vi "Tx Buffered Packet Page.vi"(8 "error in (no error)":errorcluster, 11 "Node Ptr":T5 format="%.0x") -> (0 "error out":errorcluster)   [LabVIEW 2016, in "UDP-Custom-Device System Explorer.lvlib"]
uses:
  UDP-Custom-Device System Explorer.lvlib
  Shared/Types/Shared - Transmit Flag Options.ctl
  Shared/Types/Shared - Pointer Encoding.ctl
  <vilib>/NI Veristand/Custom Device API/Custom Device Item Ref.ctl
  Shared/Types/Shared - Buffer Options.ctl
  Shared/Types/Shared - Transmit Echo Options.ctl
  Types/Page References/Refs - Tx Buffered Data Packet Page.ctl
  <vilib>/NI VeriStand/Custom Device API/Custom Device API.lvlib
  Property Accessors/Shared Packet Accessors.lvlib
  Property Accessors/Tx Packet Accessors.lvlib
  Property Accessors/Buffered Data Packet.lvlib
  Shared/UDP-Custom-Device Shared.lvlib
panel:
  in  "Debug Mode":bool caption="Auto-Assign Local NIC"
  in  "Transmit Echo Options":T1
  in  "Buffer Options":T2
  in  "Transmit Options":T3=enum."One-Shot"
  in  "Port as Channel?":bool caption="Auto-Assign Local NIC"
  in  "Pointer Encoding":T4
  in  "TTL":u16=1
  in  "Multicast?":bool caption="Auto-Assign Local NIC"
  in  "External Buffer?":bool
  in  "Buffer Size (bytes)":u32
  in  "General Header 3":cluster{"Section Name":string}={"Section Name"="Buffer Configuration"}
  in  "Prepend\nHeader?":bool caption="Auto-Assign Local NIC"
  in  "Auto-Assign Local NIC":bool
  in  "Port":u16
  in  "IP Address of Local NIC":string
  in  "Decimation":u16
  in  "General Header 2":cluster{"Section Name":string}={"Section Name"="Network Settings"}
  in  "Destination Port":u16
  in  "IP Address of Destination":string
  in  "Configure Header":bool
  in  "Endianness":u16(ring) items=["big-endian"=0, "little-endian"=2]
  out "Packet ID":i32
  in  "Description":string
  in  "Name":string
  in  "SHDocVw.IWebBrowser":refnum<k7>(container)
  in  "General Header":cluster{"Section Name":string}={"Section Name"="Buffered Transmit Packet"}
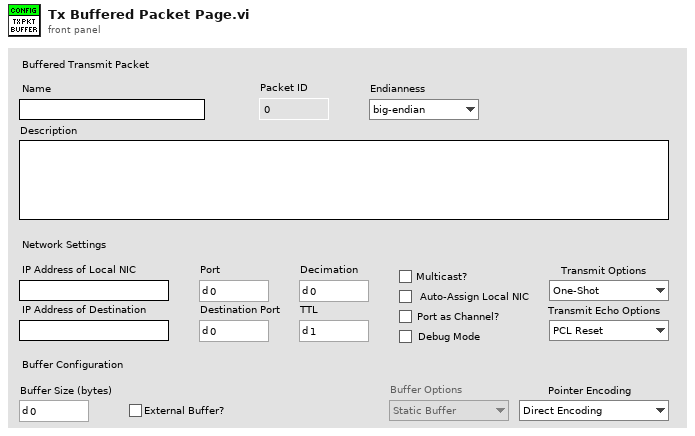
[diagram p1: front panel]
types:
  T1 = typedef "UDP-Custom-Device Shared.lvlib/Shared - Transmit Echo Options.ctl" = enum16{"PCL Reset", "Counter", "Mirror"}
  T2 = typedef "UDP-Custom-Device Shared.lvlib/Shared - Buffer Options.ctl" = enum16{"Static Buffer", "Circular Buffer"}
  T3 = typedef "UDP-Custom-Device Shared.lvlib/Shared - Transmit Flag Options.ctl" = enum16{"Always", "One-Shot", "Toggle"}
  T4 = typedef "UDP-Custom-Device Shared.lvlib/Shared - Pointer Encoding.ctl" = enum16{"Direct Encoding", "Conversion Encoding"}
  T5 = typedef "Custom Device API.lvlib/Custom Device Item Ref.ctl" = u64
  T6 = typedef "UDP-Custom-Device System Explorer.lvlib/Refs - Tx Buffered Data Packet Page.ctl" = cluster{"Name":refnum<vi>, "Description":refnum<vi>, "Packet ID":refnum<vi>, "Endianness":refnum<vi>, "Prepend\nHeader?":refnum<vi>, "Configure Header":refnum<vi>, "Decimation":refnum<vi>, "IP Address of Local NIC":refnum<vi>, "Port":refnum<vi>, "IP Address of Destination":refnum<vi>, "Destination Port":refnum<vi>, "Auto-Assign Local NIC":refnum<vi>, "External Buffer?":refnum<vi>, "Buffer Size (bytes)":refnum<vi>, "Multicast?":refnum<vi>, "TTL":refnum<vi>, "Pointer Encoding":refnum<vi>, "Port as Channel?":refnum<vi>, "Transmit Options":refnum<vi>, "Buffer Options":refnum<vi>, "Transmit Echo Options":refnum<vi>, "Debug Mode":refnum<vi>}
  T7 = enum8{"Enabled", "Disabled", "Disabled and Grayed Out"}
  T8 = typedef "Custom Device API.lvlib/Custom Device Commands.ctl" = enum16{"Default", "Item renamed", "Shutdown", "Dynamic button pressed"}
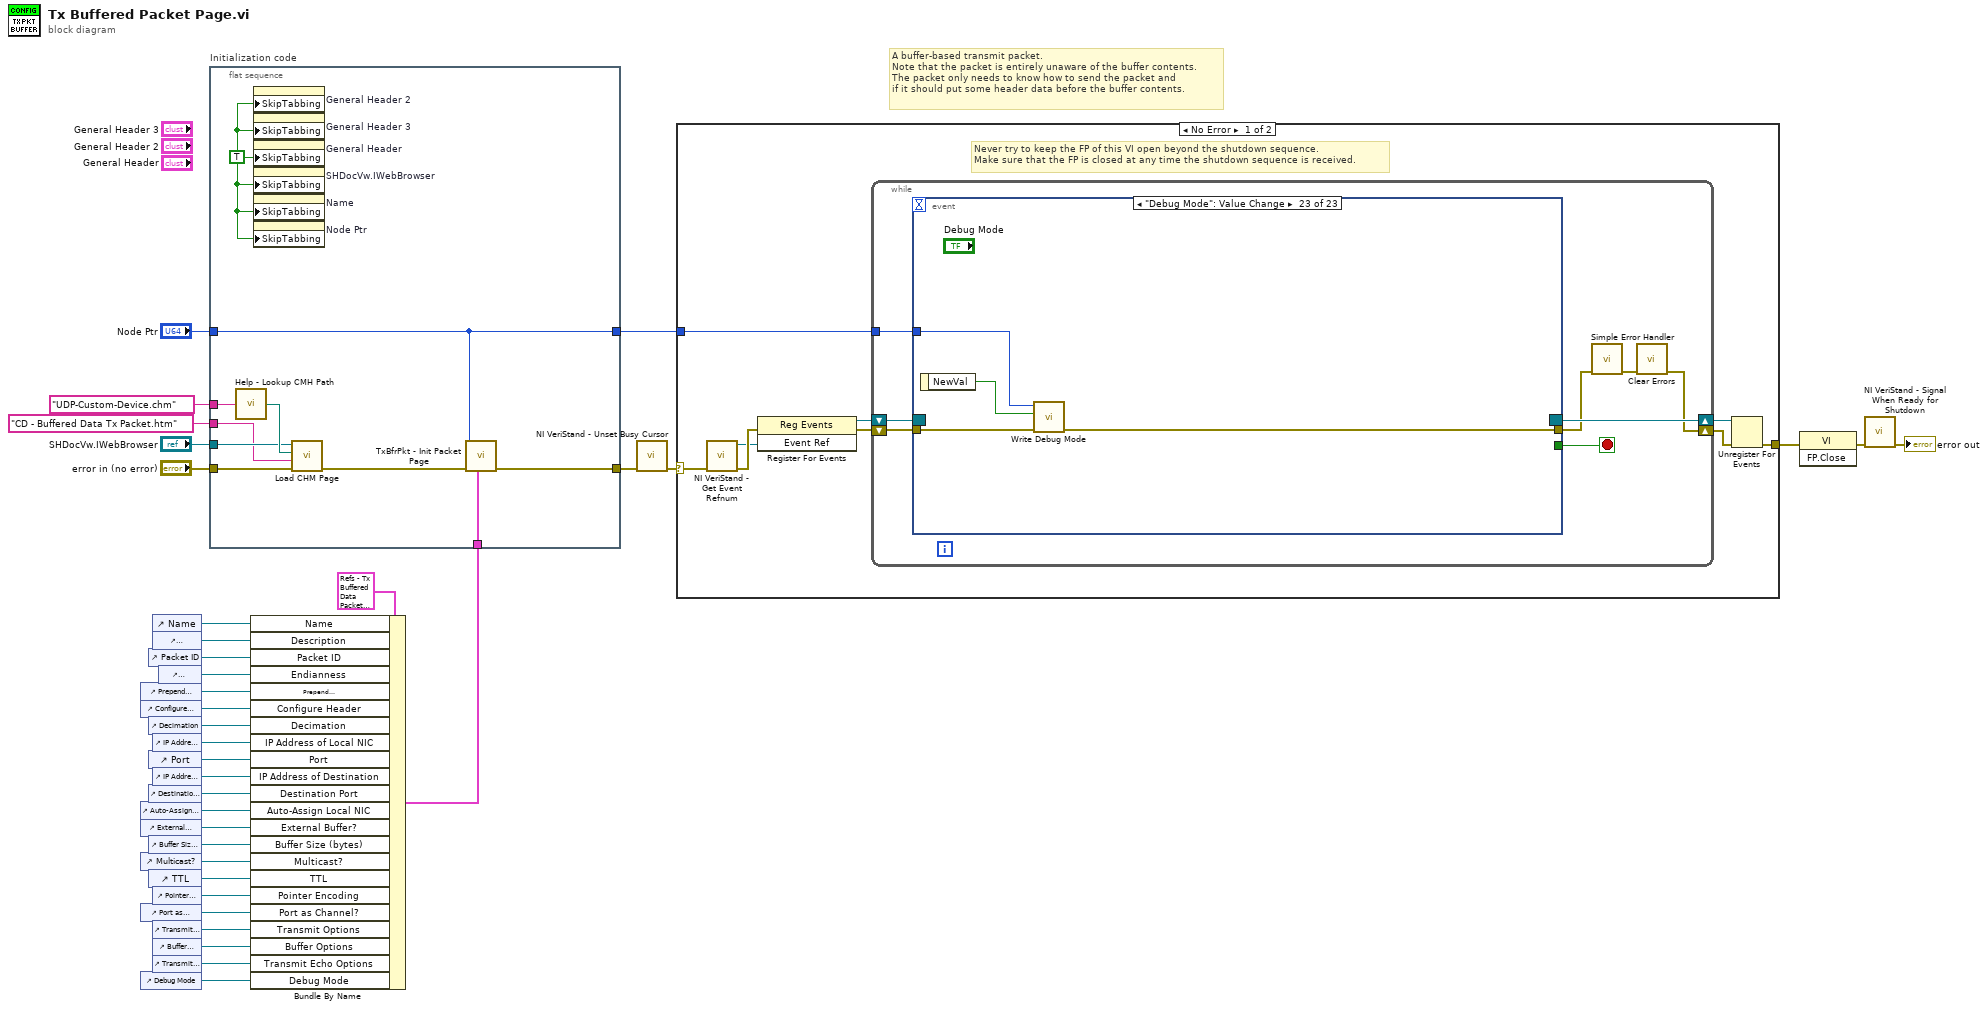
[diagram p0: block diagram]
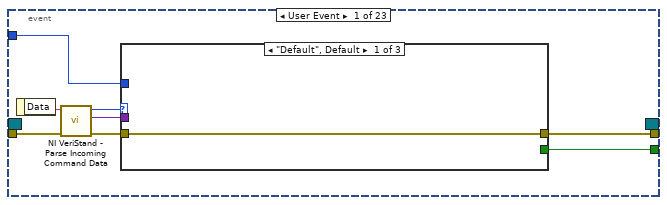
[diagram p2: hidden frame]
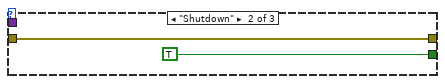
[diagram p3: hidden frame]
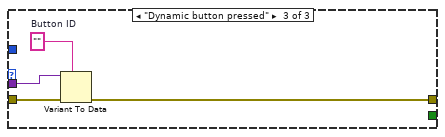
[diagram p4: hidden frame]
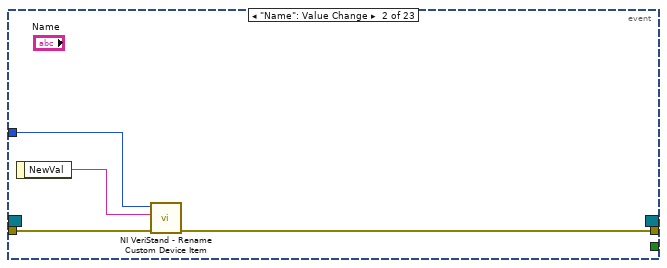
[diagram p5: hidden frame]
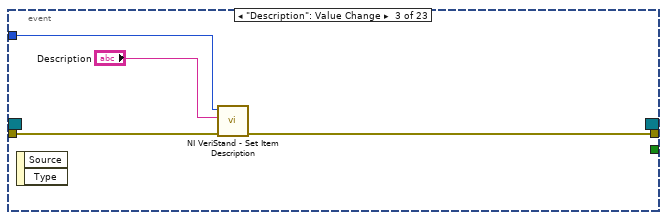
[diagram p6: hidden frame]
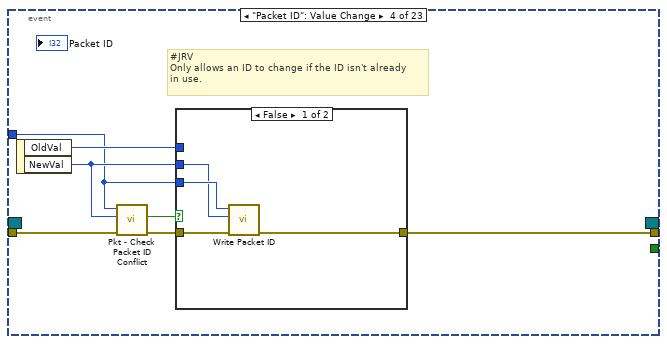
[diagram p7: hidden frame]
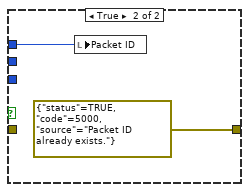
[diagram p8: hidden frame]
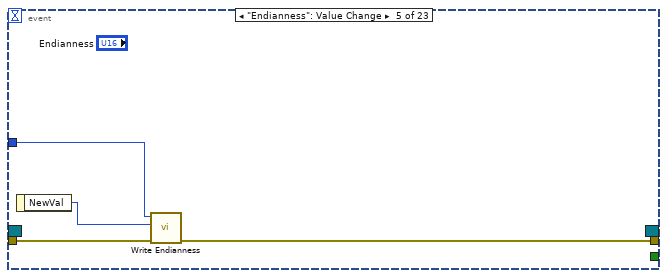
[diagram p9: hidden frame]
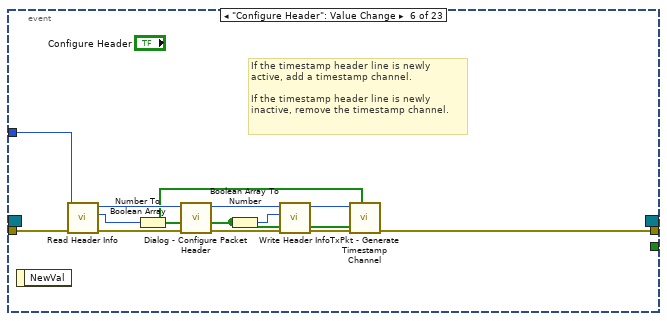
[diagram p10: hidden frame]
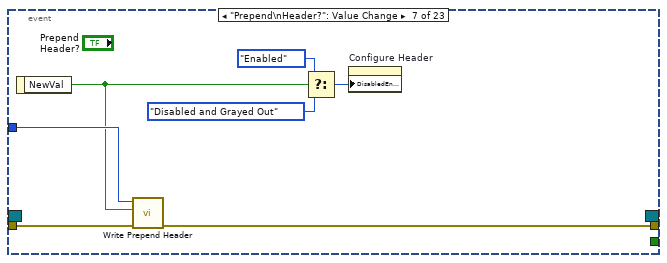
[diagram p11: hidden frame]
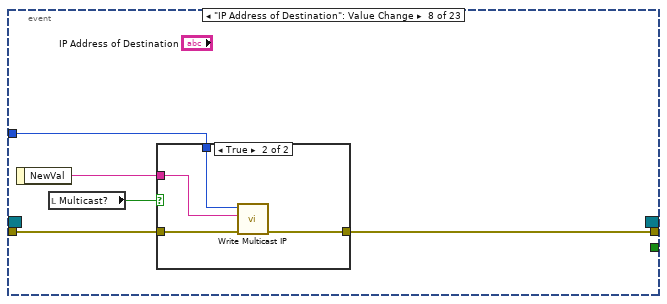
[diagram p12: hidden frame]
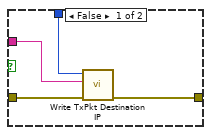
[diagram p13: hidden frame]
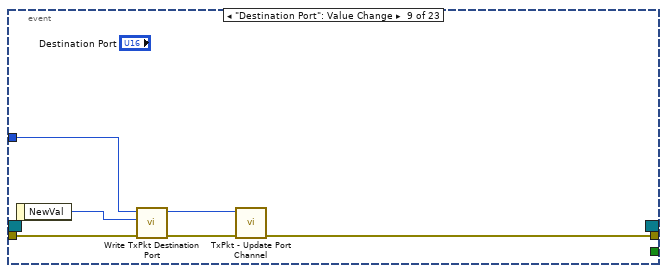
[diagram p14: hidden frame]
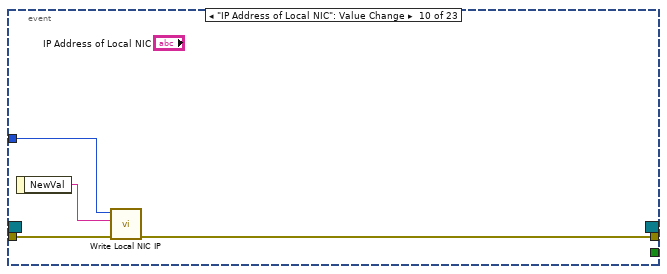
[diagram p15: hidden frame]
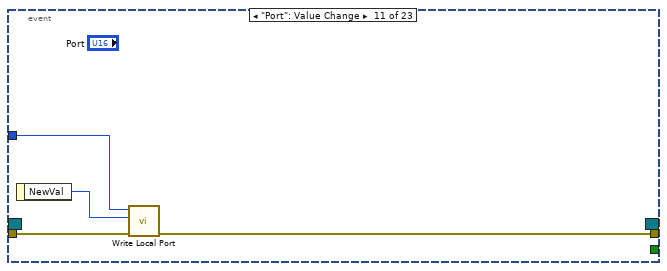
[diagram p16: hidden frame]
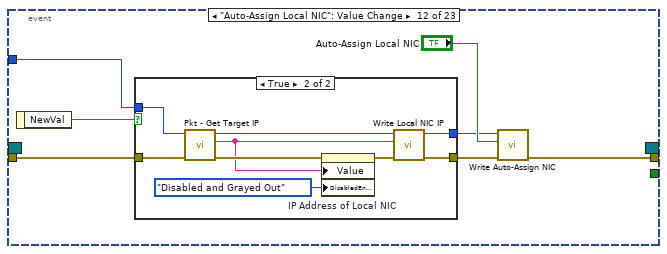
[diagram p17: hidden frame]
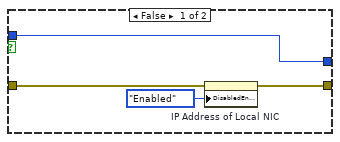
[diagram p18: hidden frame]
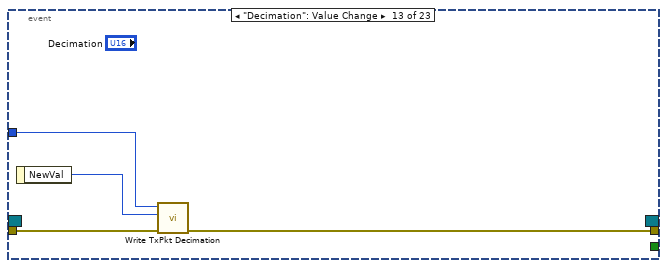
[diagram p19: hidden frame]
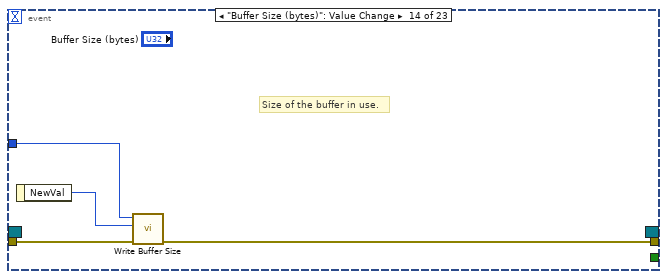
[diagram p20: hidden frame]
diagram:
  # "A buffer-based transmit packet.\nNote that the packet is entirely unaware of the buffer contents.\nThe packet only needs to know how to send the packet and\nif it should put some header data before the buffer contents."
  n1 = control-ref of="Prepend\nHeader?"() -> (w19:refnum<vi>)
  n2 = control-ref of="Configure Header"() -> (w18:refnum<vi>)
  n3 = control-ref of="Auto-Assign Local NIC"() -> (w12:refnum<vi>)
  n4 = control-ref of="External Buffer?"() -> (w11:refnum<vi>)
  n5 = control-ref of="Multicast?"() -> (w8:refnum<vi>)
  n6 = control-ref of="Port as Channel?"() -> (w5:refnum<vi>)
  n7 = control-ref of="Debug Mode"() -> (w1:refnum<vi>)
  n8 = control-ref of="Packet ID"() -> (w21:refnum<vi>)
  n9 = control-ref of="Decimation"() -> (w17:refnum<vi>)
  n10 = control-ref of="Port"() -> (w15:refnum<vi>)
  n11 = control-ref of="Destination Port"() -> (w13:refnum<vi>)
  n12 = control-ref of="Buffer Size (bytes)"() -> (w10:refnum<vi>)
  n13 = control-ref of="TTL"() -> (w7:refnum<vi>)
  n14 = control-ref of="Name"() -> (w23:refnum<vi>)
  n15 = control-ref of="Description"() -> (w22:refnum<vi>)
  n16 = control-ref of="IP Address of Local NIC"() -> (w16:refnum<vi>)
  n17 = control-ref of="IP Address of Destination"() -> (w14:refnum<vi>)
  n18 = control-ref of="Pointer Encoding"() -> (w6:refnum<vi>)
  n19 = control-ref of="Transmit Options"() -> (w4:refnum<vi>)
  n20 = control-ref of="Buffer Options"() -> (w3:refnum<vi>)
  n21 = control-ref of="Transmit Echo Options"() -> (w2:refnum<vi>)
  n22 = control-ref of="Endianness"() -> (w20:refnum<vi>)
  n23 = flat-sequence "Initialization code" {
    tunnel: "error in (no error)" -> [w44]
    tunnel: "Node Ptr" -> [w39]
    tunnel: [w37] -> w31
    tunnel: [w39] -> w28
    tunnel: "SHDocVw.IWebBrowser" -> [w43]
    tunnel: "CD - Buffered Data Tx Packet.htm" ("CD_CHM_Section") -> [w41]
    tunnel: "UDP-Custom-Device.chm" ("CD_CHM_FileName") -> [w42]
    tunnel: w9 -> [w36]
    frame #0 {
      w40 = TRUE ("Skip When Tabbing")
      n24 = call "Help - Lookup CMH Path.vi"("Main CMH File"=w42) -> ("Compiled CMH Path"=w45:path)
      n25 = property on="General Header 2" class="Clust (strict)"("SkipTabbing"=w40) -> ()  [unwired: 2 in, 2 out]
      n26 = property on="General Header 3" class="Clust (strict)"("SkipTabbing"=w40) -> ()  [unwired: 2 in, 2 out]
      n27 = property on="General Header" class="Clust (strict)"("SkipTabbing"=w40) -> ()  [unwired: 2 in, 2 out]
      n28 = property on="SHDocVw.IWebBrowser" class="AXCont"("SkipTabbing"=w40) -> ()  [unwired: 2 in, 2 out]
      n29 = property on="Name" class="Str"("SkipTabbing"=w40) -> ()  [unwired: 2 in, 2 out]
      n30 = property on="Node Ptr" class="DigNum (strict)"("SkipTabbing"=w40) -> ()  [unwired: 2 in, 2 out]
      n31 = call <vilib>:"Load CHM Page.vi"("error in (no error)"=w44, "HTML File"=w41, "Compiled CHM Path"=w45, "Web Browser Reference"=w43) -> ("error out"=w38:errorcluster)  [unwired: 7 in]
      n32 = call "TxBfrPkt - Init Packet Page.vi"("Tx Buffered Data Packet Refs"=w36, "error in (no error)"=w38, "Node Ptr In"=w39) -> ("error out"=w37:errorcluster)  [unwired: 7 in, 1 out]
    }
  }
  n33 = Bundle By Name(cluster=T6 {"Name"=refnum, "Description"=refnum, "Packet ID"=refnum, "Endianness"=refnum, "Prepend\nHeader?"=refnum, "Configure Header"=refnum, "Decimation"=refnum, "IP Address of Local NIC"=refnum, "Port"=refnum, "IP Address of Destination"=refnum, "Destination Port"=refnum, "Auto-Assign Local NIC"=refnum, "External Buffer?"=refnum, "Buffer Size (bytes)"=refnum, "Multicast?"=refnum, "TTL"=refnum, "Pointer Encoding"=refnum, "Port as Channel?"=refnum, "Transmit Options"=refnum, "Buffer Options"=refnum, "Transmit Echo Options"=refnum, "Debug Mode"=refnum} ("Tx Buffered Data Packet Refs"), "Name"=w23, "Description"=w22, "Packet ID"=w21, "Endianness"=w20, "Prepend\nHeader?"=w19, "Configure Header"=w18, "Decimation"=w17, "IP Address of Local NIC"=w16, "Port"=w15, "IP Address of Destination"=w14, "Destination Port"=w13, "Auto-Assign Local NIC"=w12, "External Buffer?"=w11, "Buffer Size (bytes)"=w10, "Multicast?"=w8, "TTL"=w7, "Pointer Encoding"=w6, "Port as Channel?"=w5, "Transmit Options"=w4, "Buffer Options"=w3, "Transmit Echo Options"=w2, "Debug Mode"=w1) -> (w9:T6)
  n34 = call <vilib>:"NI VeriStand - Unset Busy Cursor.vi"("error in (no error)"=w31) -> ("error out"=w30:errorcluster)  [unwired: 10 out]
  n35 = case shown="No Error" w30 {
    selector: w30 -> [w46 w233]
    tunnel: [w51 w231] -> w35
    tunnel: w28 -> [w47 _]
    frame No Error {
      # "Never try to keep the FP of this VI open beyond the shutdown sequence.\nMake sure that the FP is closed at any time the shutdown sequence is received."
      n36 = call <vilib>:"NI VeriStand - Get Event Refnum.vi"("error in (no error)"=w46) -> ("error out"=w54:errorcluster, "Event Ref"=w50:refnum<user-event>)  [unwired: 9 out]
      n37 = register-events(error in=w54, w50) -> (reference out=w48:refnum<event-registration>, error out=w49:errorcluster)  [unwired: 1 in]
      n38 = while {
        tunnel: w47 -> [w58]
        shift-right: [w55] -> w52
        shift-left: w49 -> [w61]
        shift-right: [w62] -> w53
        shift-left: w48 -> [w60]
        stop <- w59 stop-if-true
        n39 = event shown="[22] \"Debug Mode\": Value Change" {
          selector: w60 -> [_ _ _ _ _ _ _ _ _ _ _ _ _ _ _ _ _ _ _ _ _ _ _]
          dyn-events: [_ _ _ _ _ _ _ _ _ _ _ _ _ _ _ _ _ _ _ _ _ _ _] -> w62
          timeout: _ -> [_ _ _ _ _ _ _ _ _ _ _ _ _ _ _ _ _ _ _ _ _ _ _]
          tunnel: w61 -> [w70 w81 w85 w90 w102 w105 w119 w125 w141 w143 w149 w156 w173 w175 w182 w185 w193 w207 w214 w217 w222 w225 w228]
          tunnel: [w66 _ _ _ _ _ _ _ _ _ _ _ _ _ _ _ _ _ _ _ _ _ _] -> w59
          tunnel: [w65 w79 w82 w86 w99 w103 w116 w124 w136 w142 w146 w151 w170 w174 w179 w184 w188 w205 w209 w215 w219 w223 w227] -> w57
          tunnel: w58 -> [w64 w80 w84 w87 w101 w104 w118 w127 w139 w144 w147 w154 w172 w177 w183 w186 w194 w208 w212 w218 w221 w226 w230]
          event User Event {
            n40 = event-data() -> ("Data"=w69:string)  [unwired: 1 out]
            n41 = call <vilib>:"NI VeriStand - Parse Incoming Command Data.vi"("error in (no error)"=w70, "Incoming data"=w69) -> ("error out"=w68:errorcluster, "Outgoing data"=w63:variant, "Action"=w67:T8)  [unwired: 7 out]
            n42 = case shown="\"Default\", Default" w67 {
              tunnel: w68 -> [w71 w72 w77]
              tunnel: [_ TRUE _] -> w66
              tunnel: [w71 w72 w74] -> w65
              tunnel: w64 -> [_ _ _]
              tunnel: w63 -> [_ _ w76]
              frame "Default", Default {
              }
              frame "Shutdown" {
              }
              frame "Dynamic button pressed" {
                w75 = ""  # Button ID
                n43 = Variant To Data(error in=w77, type=w75, Variant=w76) -> (error out=w74:errorcluster)  [unwired: 1 out]
              }
            }
          }
          event "Name": Value Change {
            n44 = event-data() -> ("NewVal"=w78:string)  [unwired: 1 out]
            n45 = call <vilib>:"NI VeriStand - Rename Custom Device Item.vi"("error in (no error)"=w81, "New Name"=w78, "Item Ref in"=w80) -> ("error out"=w79:errorcluster)  [unwired: 6 in, 2 out]
          }
          event "Description": Value Change {
            n46 = event-data() -> ()  [unwired: 3 out]
            n47 = call <vilib>:"NI VeriStand - Set Item Description.vi"("error in (no error)"=w85, "Description"="Description", "Item Ref in"=w84) -> ("error out"=w82:errorcluster)  [unwired: 6 in, 2 out]
          }
          event "Packet ID": Value Change {
            # "#JRV\nOnly allows an ID to change if the ID isn't already\nin use."
            n48 = event-data() -> ("OldVal"=w89:i32, "NewVal"=w88:i32)  [unwired: 1 out]
            n49 = call "Pkt - Check Packet ID Conflict.vi"("error in (no error)"=w90, "New ID"=w88, "Packet Ref In"=w87) -> ("error out"=w92:errorcluster, "Conflicting ID?"=w91:bool)  [unwired: 7 in]
            n50 = case shown="False" w91 {
              tunnel: w92 -> [w94 _]
              tunnel: w87 -> [w96 _]
              tunnel: [w93 errorcluster {"status"=TRUE, "code"=5000, "source"="Packet ID already exists."} ("error out")] -> w86
              tunnel: w89 -> [_ w97]
              tunnel: w88 -> [w95 _]
              frame False {
                n51 = call "Write Packet ID.vi"("error in (no error)"=w94, "Packet ID"=w95, "Node Ptr"=w96) -> ("error out"=w93:errorcluster)  [unwired: 7 in, 1 out]
              }
              frame True {
                n52 = local write "Packet ID"(w97) -> ()
              }
            }
          }
          event "Endianness": Value Change {
            n53 = event-data() -> ("NewVal"=w100:u16)  [unwired: 1 out]
            n54 = call "Write Endianness.vi"("error in (no error)"=w102, "Endianness"=w100, "Node Ptr"=w101) -> ("error out"=w99:errorcluster)  [unwired: 7 in, 1 out]
          }
          event "Configure Header": Value Change {
            # "If the timestamp header line is newly\nactive, add a timestamp channel.\n\nIf the timestamp header line is newly\ninactive, remove the timestamp channel."
            n55 = event-data() -> ()  [unwired: 2 out]
            n56 = call "Read Header Info.vi"("error in (no error)"=w105, "Node Ptr"=w104) -> ("error out"=w113:errorcluster, "Header Info"=w114:u32, "Node Ptr out"=w115:T5)  [unwired: 7 in]
            n57 = Number To Boolean Array(number=w114) -> (Boolean array=w106:bool[])
            n58 = call "Dialog - Configure Packet Header.vi"("error in (no error)"=w113, "Header Elements In"=w106, "Packet Ref in"=w115) -> ("error out"=w109:errorcluster, "Header Elements Out"=w107:bool[], "Packet Ref out"=w108:T5)  [unwired: 6 in]
            n59 = Boolean Array To Number(Boolean array=w107) -> (number=w110:u32)
            n60 = call "Write Header Info.vi"("error in (no error)"=w109, "Header Info"=w110, "Node Ptr"=w108) -> ("error out"=w112:errorcluster, "Node Ptr out"=w111:T5)  [unwired: 7 in]
            n61 = call "TxPkt - Generate Timestamp Channel.vi"("New Header Config"=w107, "Previous Header Config"=w106, "error in (no error)"=w112, "Packet Ref in"=w111) -> ("error out"=w103:errorcluster)  [unwired: 6 in, 1 out]
          }
          event "Prepend\nHeader?": Value Change {
            n62 = event-data() -> ("NewVal"=w117:bool)  [unwired: 1 out]
            n63 = call "Write Prepend Header.vi"("error in (no error)"=w119, "Prepend Header"=w117, "Node Ptr"=w118) -> ("error out"=w116:errorcluster)  [unwired: 7 in, 1 out]
            n64 = Select(t=T7."Enabled" ("Disabled"), s=w117, f=T7."Disabled and Grayed Out" ("Disabled")) -> (s? t:f=w120:T7)
            n65 = property on="Configure Header" class="Bool"("DisabledEnum"=w120) -> ()  [unwired: 2 in, 2 out]
          }
          event "IP Address of Destination": Value Change {
            n66 = event-data() -> ("NewVal"=w126:string)  [unwired: 1 out]
            n67 = local read "Multicast?"() -> (w123:bool)
            n68 = case shown="True" w123 {
              tunnel: w127 -> [w131 w135]
              tunnel: w126 -> [w130 w132]
              tunnel: w125 -> [w129 w134]
              tunnel: [w128 w133] -> w124
              frame False {
                n69 = call "Write TxPkt Destination IP.vi"("error in (no error)"=w129, "Destination IP"=w130, "Node Ptr"=w131) -> ("error out"=w128:errorcluster)  [unwired: 7 in, 1 out]
              }
              frame True {
                n70 = call "Write Multicast IP.vi"("error in (no error)"=w134, "Multicast IP Address"=w132, "Node Ptr"=w135) -> ("error out"=w133:errorcluster)  [unwired: 7 in, 1 out]
              }
            }
          }
          event "Destination Port": Value Change {
            n71 = event-data() -> ("NewVal"=w140:u16)  [unwired: 1 out]
            n72 = call "Write TxPkt Destination Port.vi"("error in (no error)"=w141, "Destination Port"=w140, "Node Ptr"=w139) -> ("error out"=w137:errorcluster, "Node Ptr out"=w138:T5)  [unwired: 7 in]
            n73 = call "TxPkt - Update Port Channel.vi"("error in (no error)"=w137, "Packet Ref in"=w138) -> ("error out"=w136:errorcluster)  [unwired: 8 in, 1 out]
          }
          event "IP Address of Local NIC": Value Change {
            n74 = event-data() -> ("NewVal"=w145:string)  [unwired: 1 out]
            n75 = call "Write Local NIC IP.vi"("error in (no error)"=w143, "IP Address of Local NIC"=w145, "Node Ptr"=w144) -> ("error out"=w142:errorcluster)  [unwired: 7 in, 1 out]
          }
          event "Port": Value Change {
            n76 = event-data() -> ("NewVal"=w148:u16)  [unwired: 1 out]
            n77 = call "Write Local Port.vi"("error in (no error)"=w149, "Port"=w148, "Node Ptr"=w147) -> ("error out"=w146:errorcluster)  [unwired: 7 in, 1 out]
          }
          event "Auto-Assign Local NIC": Value Change {
            n78 = event-data() -> ("NewVal"=w155:bool)  [unwired: 1 out]
            n79 = case shown="True" w155 {
              tunnel: w156 -> [w160 w167]
              tunnel: [w158 w162] -> w150
              tunnel: [w157 w161] -> w152
              tunnel: w154 -> [w157 w166]
              frame False {
                n80 = property on="IP Address of Local NIC" class="Str"(error in=w160, "DisabledEnum"=T7."Enabled" ("Disabled")) -> (error out=w158:errorcluster)  [unwired: 1 in, 1 out]
              }
              frame True {
                n81 = call "Pkt - Get Target IP.vi"("error in"=w167, "Item Ref in"=w166) -> ("error out"=w169:errorcluster, "IPAddress"=w164:string, "Item Ref out"=w165:T5)  [unwired: 7 in]
                n82 = property on="IP Address of Local NIC" class="Str"(error in=w169, "Value"=w164, "DisabledEnum"=T7."Disabled and Grayed Out" ("Disabled")) -> (error out=w163:errorcluster)  [unwired: 1 in, 1 out]
                n83 = call "Write Local NIC IP.vi"("error in (no error)"=w163, "IP Address of Local NIC"=w164, "Node Ptr"=w165) -> ("error out"=w162:errorcluster, "Node Ptr out"=w161:T5)  [unwired: 7 in]
              }
            }
            n84 = call "Write Auto-Assign NIC.vi"("error in (no error)"=w150, "Auto-Assign NIC"="Auto-Assign Local NIC", "Node Ptr"=w152) -> ("error out"=w151:errorcluster)  [unwired: 7 in, 1 out]
          }
          event "Decimation": Value Change {
            n85 = event-data() -> ("NewVal"=w171:u16)  [unwired: 1 out]
            n86 = call "Write TxPkt Decimation.vi"("error in (no error)"=w173, "Decimation"=w171, "Node Ptr"=w172) -> ("error out"=w170:errorcluster)  [unwired: 7 in, 1 out]
          }
          event "Buffer Size (bytes)": Value Change {
            # "Size of the buffer in use."
            n87 = event-data() -> ("NewVal"=w176:u32)  [unwired: 1 out]
            n88 = call "Write Buffer Size.vi"("error in (no error)"=w175, "Buffer Size"=w176, "Node Ptr"=w177) -> ("error out"=w174:errorcluster)  [unwired: 7 in, 1 out]
          }
          event "External Buffer?": Value Change {
            # "Change the buffer channel to an input (external) or output (internal) channel."
            n89 = event-data() -> ("NewVal"=w178:bool)  [unwired: 1 out]
            n90 = call "Write External Buffer.vi"("error in (no error)"=w182, "External Buffer"=w178, "Node Ptr"=w183) -> ("error out"=w180:errorcluster, "Node Ptr out"=w181:T5)  [unwired: 7 in]
            n91 = call "BfrPkt - Set Buffer Direction.vi"("error in (no error)"=w180, "External?"=w178, "Node Ptr"=w181) -> ("error out"=w179:errorcluster)  [unwired: 7 in, 1 out]
          }
          event "TTL": Value Change {
            n92 = event-data() -> ("NewVal"=w187:u16)  [unwired: 1 out]
            n93 = call "Write TTL.vi"("error in (no error)"=w185, "TTL"=w187, "Node Ptr"=w186) -> ("error out"=w184:errorcluster)  [unwired: 7 in, 1 out]
          }
          event "Multicast?": Value Change {
            n94 = event-data() -> ("NewVal"=w192:bool)  [unwired: 1 out]
            n95 = call "Write Multicast.vi"("error in (no error)"=w193, "Multicast"=w192, "Node Ptr"=w194) -> ("error out"=w190:errorcluster, "Node Ptr out"=w191:T5)  [unwired: 7 in]
            n96 = case shown="True" w192 {
              tunnel: [w199 w200] -> w188
              tunnel: [w198 w201] -> w189
              tunnel: [w197 w202] -> _
              tunnel: w191 -> [w196 w204]
              tunnel: w190 -> [w195 w203]
              frame False {
                n97 = call "Read TxPkt Destination IP.vi"("error in (no error)"=w195, "Node Ptr"=w196) -> ("error out"=w199:errorcluster, "Destination IP"=w198:string, "Node Ptr out"=w197:T5)  [unwired: 7 in]
              }
              frame True {
                n98 = call "Read Multicast IP.vi"("error in (no error)"=w203, "Node Ptr"=w204) -> ("error out"=w200:errorcluster, "Multicast IP Address"=w201:string, "Node Ptr out"=w202:T5)  [unwired: 7 in]
              }
            }
            n99 = local write "IP Address of Destination"(w189) -> ()
          }
          event Value Change {
            n100 = event-data() -> ("NewVal"=w206:T4)  [unwired: 1 out]
            n101 = call "Write Pointer Encoding.vi"("error in (no error)"=w207, "Pointer Encoding"=w206, "Node Ptr"=w208) -> ("error out"=w205:errorcluster)  [unwired: 7 in, 1 out]
          }
          event "Port as Channel?": Value Change {
            n102 = event-data() -> ("NewVal"=w213:bool)  [unwired: 1 out]
            n103 = call "Write TxPkt Port as Channel.vi"("error in (no error)"=w214, "Port as Channel"=w213, "Node Ptr"=w212) -> ("error out"=w210:errorcluster, "Node Ptr out"=w211:T5)  [unwired: 7 in]
            n104 = call "TxPkt - Handle Port Channel.vi"("error in (no error)"=w210, "Packet Ref in"=w211) -> ("error out"=w209:errorcluster)  [unwired: 8 in, 1 out]
          }
          event Value Change {
            n105 = event-data() -> ("NewVal"=w216:T3)  [unwired: 1 out]
            n106 = call "Write TxPkt Transmit Option.vi"("error in (no error)"=w217, "Transmit Options"=w216, "Node Ptr"=w218) -> ("error out"=w215:errorcluster)  [unwired: 7 in, 1 out]
          }
          event Value Change {
            n107 = event-data() -> ("NewVal"=w220:T2)  [unwired: 1 out]
            n108 = call "Write Buffer Option.vi"("error in (no error)"=w222, "Buffer Option"=w220, "Node Ptr"=w221) -> ("error out"=w219:errorcluster)  [unwired: 7 in, 1 out]
          }
          event Value Change {
            n109 = event-data() -> ("NewVal"=w224:T1)  [unwired: 1 out]
            n110 = call "Write TxPkt Transmit Echo Option.vi"("error in (no error)"=w225, "Transmit Echo Options"=w224, "Node Ptr"=w226) -> ("error out"=w223:errorcluster)  [unwired: 7 in, 1 out]
          }
          event "Debug Mode": Value Change {
            n111 = event-data() -> ("NewVal"=w229:bool)  [unwired: 1 out]
            n112 = call "Write Debug Mode.vi"("error in (no error)"=w228, "Debug Mode"=w229, "Node Ptr"=w230) -> ("error out"=w227:errorcluster)  [unwired: 7 in, 1 out]
          }
        }
        n113 = call <vilib>:"Simple Error Handler.vi"("error in (no error)"=w57) -> ("error out"=w56:errorcluster)  [unwired: 1 in, 7 out]
        n114 = call <vilib>:"Clear Errors.vi"("error in (no error)"=w56) -> ("error out"=w55:errorcluster)  [unwired: 1 in, 5 out]
      }
      n115 = Unregister For Events(event registration refnum=w53, error in=w52) -> (error out=w51:errorcluster)
    }
    frame Error {
      n116 = call <vilib>:"Simple Error Handler.vi"("error in (no error)"=w233) -> ("error out"=w232:errorcluster)  [unwired: 1 in, 7 out]
      n117 = call <vilib>:"Clear Errors.vi"("error in (no error)"=w232) -> ("error out"=w231:errorcluster)  [unwired: 1 in, 5 out]
    }
  }
  n118 = invoke class="VI" method="FP.Close"(error in=w35) -> (error out=w34:errorcluster)  [unwired: 2 in, 2 out]
  n119 = call <vilib>:"NI VeriStand - Signal When Ready for Shutdown.vi"("error in (no error)"=w34) -> ("error out"=→"error out":errorcluster)  [unwired: 10 out]
